vi "Check Amount of Pyramid Levels.vi"(8 "error in (no error)":errorcluster, 11 "Refnum in":T1) -> (0 "error out":errorcluster, 2 "Image Dup":T1, 3 "Pyr Levels":i32)   [LabVIEW 2023]
uses:
  <vilib>/vision/Image Controls.llb/IMAQ Image.ctl
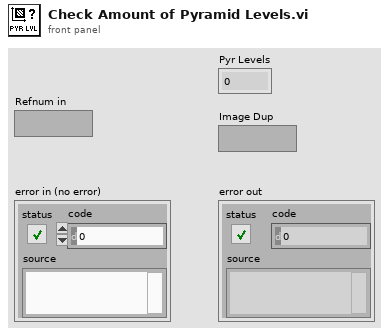
[diagram p1: front panel]
types:
  T1 = typedef "IMAQ Image.ctl" = refnum<image>
  T2 = typedef "Image Type" = u32
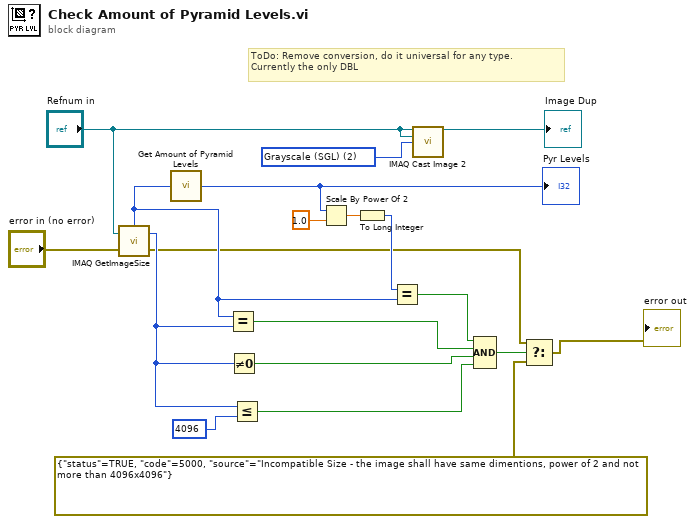
[diagram p0: block diagram]
diagram:
  w1 = T2 2 items=["Grayscale (U8)", "Grayscale (I16)", "Grayscale (SGL)", "Complex (CSG)", "RGB (U32)", "HSL (U32)", "RGB (U64)", "Grayscale (U16)"] ("Image Type")
  # "ToDo: Remove conversion, do it universal for any type.\nCurrently the only DBL"
  n1 = call "IMAQ GetImageSize"("Image"="Refnum in", "error in (no error)"="error in (no error)") -> ("Y Resolution"=w15:i32, "X Resolution"=w12:i32, "error out"=w6:errorcluster)  [unwired: 2 in]
  n2 = call "Get Amount of Pyramid Levels.vi"("X Resolution"=w12) -> ("Pyr Levels"=w17:i32)
  "Pyr Levels" <- w17
  n3 = Equal?(x=w12, y=w15) -> (x = y?=w10:bool)
  n4 = Not Equal To 0?(x=w15) -> (x != 0?=w9:bool)
  n5 = Less Or Equal?(x=w15, y=4096) -> (x <= y?=w8:bool)
  n6 = Scale By Power Of 2(n=w17, x=1.0) -> (x*2^n=w16:dbl)
  n7 = To Long Integer(number=w16) -> (32bit integer=w13:i32)
  n8 = Equal?(x=w13, y=w12) -> (x = y?=w11:bool)
  n9 = call "IMAQ Cast Image 2"("Image Src"="Refnum in", "Image Dst"="Refnum in", "Image Type"=w1) -> ("Image Dst Out"=→"Image Dup":T1)  [unwired: 11 in, 1 out]
  n10 = Compound Arithmetic op=AND(w11, w10, w9, w8) -> (w7:bool)
  n11 = Select(t=w6, s=w7, f=errorcluster {"status"=TRUE, "code"=5000, "source"="Incompatible Size - the image shall have same dimentions, power of 2 and not more than 4096x4096"}) -> (s? t:f=→"error out":errorcluster)
